vi "New Buffer.vi"(7 "byte order (big-endian)":T1(ring), 8 "error in (no error)":errorcluster, 9 "buffer offset":u64 format="%d bytes", 10 "buffer size":u64 format="%d bytes", 11 "Buffer type":refnum<class "Buffer.lvclass">) -> (0 "error out":errorcluster, 3 "Buffer out":refnum<class "Buffer.lvclass">)   [LabVIEW 2017, in "DSF Core.lvlib" / "Buffer.lvclass"]
uses:
  Buffer.lvclass
  Buffer.lvclass/Buffer.ctl
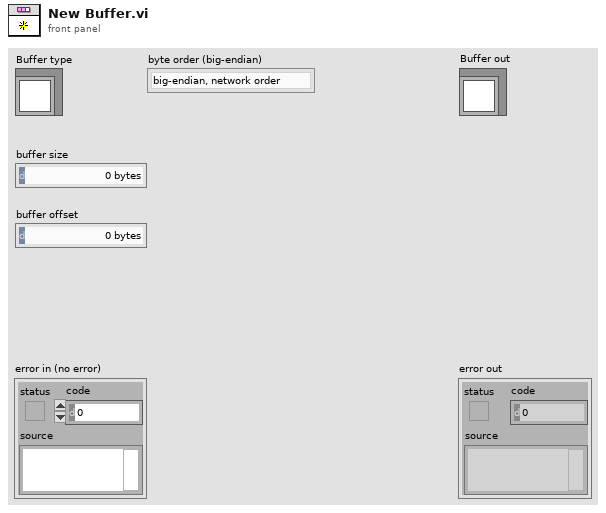
[diagram p1: front panel]
types:
  T1 = enum16{"big-endian, network order", "native, host order", "little-endian"}
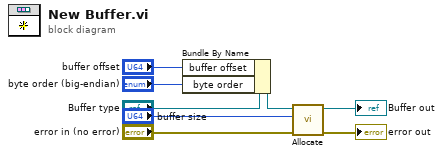
[diagram p0: block diagram]
diagram:
  n1 = Bundle By Name(cluster="Buffer type", "buffer offset"="buffer offset", "byte order"="byte order (big-endian)") -> (w5:refnum<class "Buffer.lvclass">)
  n2 = call-dynamic "Allocate.vi"("error in (no error)"="error in (no error)", "size"="buffer size", "Pointer in"=w5) -> ("error out"=→"error out":errorcluster, "Pointer out"=→"Buffer out":refnum<class "Buffer.lvclass">)  [unwired: 7 in]
